vi "TCam_WellTemp.vi"(9 "Offset":dbl, 10 "Pixels":cluster{"X":i32, "Y":i32}[][](array[cluster]), 11 "Image in":T2) -> (0 "All Pixel temps for all wells":dbl[][](array[numeric]), 1 "Mean Temp":dbl format="%0.2f", 2 "Image Out":T2, 3 "Temps":dbl[](array[numeric]), 4 "Output cluster":T1)   [LabVIEW 2024]
uses:
  <vilib>/vision/Image Controls.llb/IMAQ Image.ctl
  <vilib>/Analysis/baseanly.llb/Mean (DBL).vi
  <vilib>/vision/NI_Vision_Development_Module.lvlib
  <vilib>/Analysis/NI_AALBase.lvlib
panel:
  out "error out":errorcluster
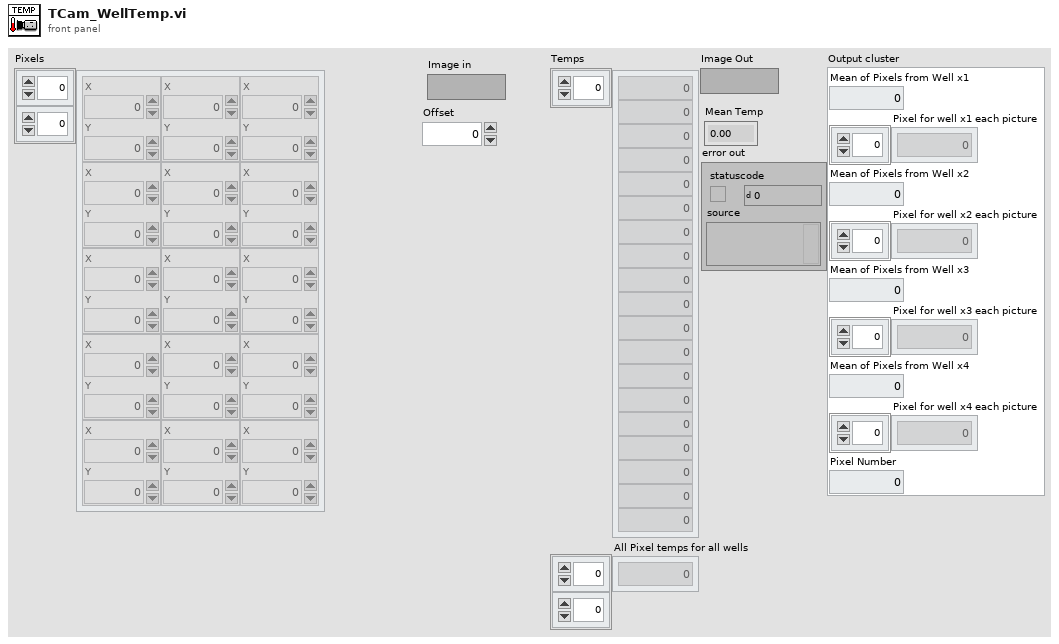
[diagram p1: front panel]
types:
  T1 = cluster{"Mean of Pixels from Well x1":dbl, "Pixel for well x1 each picture":dbl[], "Mean of Pixels from Well x2":dbl, "Pixel for well x2 each picture":dbl[], "Mean of Pixels from Well x3":dbl, "Pixel for well x3 each picture":dbl[], "Mean of Pixels from Well x4":dbl, "Pixel for well x4 each picture":dbl[], "Pixel Number":i32}
  T2 = typedef "IMAQ Image.ctl" = refnum<image>
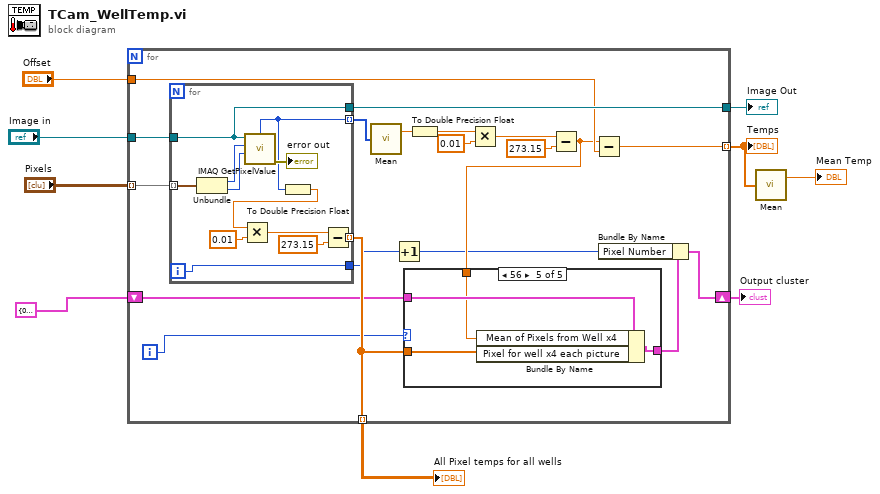
[diagram p0: block diagram]
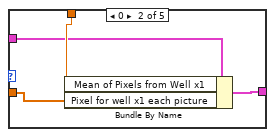
[diagram p3: hidden frame]
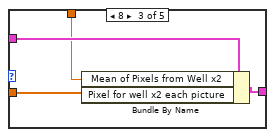
[diagram p4: hidden frame]
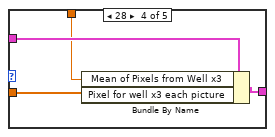
[diagram p5: hidden frame]
diagram:
  n1 = for {
    tunnel: "Image in" -> [w28]
    tunnel: "Pixels" -> [w27] mode=indexing
    tunnel: [w24] -> w6 mode=indexing
    tunnel: [w25] -> w7
    tunnel: "Offset" -> [w23]
    tunnel: [w16] -> w3 mode=indexing
    shift-right: [w13] -> w1
    shift-left: T1 {"Mean of Pixels from Well x1"=0.0, "Pixel for well x1 each picture"=[], "Mean of Pixels from Well x2"=0.0, "Pixel for well x2 each picture"=[], "Mean of Pixels from Well x3"=0.0, "Pixel for well x3 each picture"=[], "Mean of Pixels from Well x4"=0.0, "Pixel for well x4 each picture"=[], "Pixel Number"=0} ("input cluster") -> [w15]
    i -> [w10]
    n2 = for {
      tunnel: w28 -> [w54]
      tunnel: w27 -> [w57] mode=indexing
      tunnel: [w52] -> w26 mode=indexing
      tunnel: [w54] -> w25
      tunnel: [w47] -> w16 mode=indexing
      tunnel: [w46] -> w12
      i -> [w46]
      n3 = Unbundle(w57) -> ("X"=w56:i32, "Y"=w55:i32)
      n4 = call "IMAQ GetPixelValue"("Image"=w54, "X Coordinate"=w56, "Y Coordinate"=w55) -> ("Pixel Value (U16)"=w52:u16, "error out"=→"error out":errorcluster)  [unwired: 3 in, 3 out]
      n5 = To Double Precision Float(number=w52) -> (double precision float=w48:dbl)
      n6 = Multiply(x=w48, y=0.01) -> (x*y=w50:dbl)
      n7 = Subtract(x=w50, y=273.15) -> (x-y=w47:dbl)
    }
    n8 = call-poly <vilib>:"Mean.vi"("X"=w26) -> ("mean"=w18:dbl)  [unwired: 1 out]
    n9 = Increment(x=w12) -> (x+1=w11:i32)
    n10 = To Double Precision Float(number=w18) -> (double precision float=w20:dbl)
    n11 = Multiply(x=w20, y=0.01) -> (x*y=w21:dbl)
    n12 = Subtract(x=w21, y=273.15) -> (x-y=w17:dbl)
    n13 = case shown="56" w10 {
      tunnel: w16 -> [_ w30 w35 w39 w43]
      tunnel: w17 -> [_ w32 w34 w38 w42]
      tunnel: [w29 w33 w36 w40 w44] -> w14
      tunnel: w15 -> [w29 w31 w37 w41 w45]
      frame 1111, Default {
      }
      frame 0 {
        n14 = Bundle By Name(cluster=w31, "Mean of Pixels from Well x1"=w32, "Pixel for well x1 each picture"=w30) -> (w33:T1)
      }
      frame 8 {
        n15 = Bundle By Name(cluster=w37, "Mean of Pixels from Well x2"=w34, "Pixel for well x2 each picture"=w35) -> (w36:T1)
      }
      frame 28 {
        n16 = Bundle By Name(cluster=w41, "Mean of Pixels from Well x3"=w38, "Pixel for well x3 each picture"=w39) -> (w40:T1)
      }
      frame 56 {
        n17 = Bundle By Name(cluster=w45, "Mean of Pixels from Well x4"=w42, "Pixel for well x4 each picture"=w43) -> (w44:T1)
      }
    }
    n18 = Subtract(x=w17, y=w23) -> (x-y=w24:dbl)
    n19 = Bundle By Name(cluster=w14, "Pixel Number"=w11) -> (w13:T1)
  }
  "Temps" <- w6
  "Image Out" <- w7
  "All Pixel temps for all wells" <- w3
  "Output cluster" <- w1
  n20 = call-poly <vilib>:"Mean.vi"("X"=w6) -> ("mean"=→"Mean Temp":dbl)  [unwired: 1 out]
